vi "Add_Template.vi"(1 "X":dbl, 2 "Y":dbl) -> (0 "Output":dbl)   [LabVIEW 2013]
panel:
  # "Your code should take inputs X and Y and set output to the sum of X and Y"
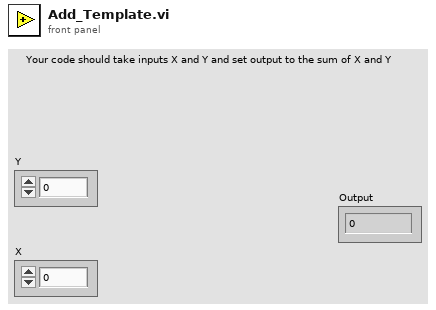
[diagram p1: front panel]
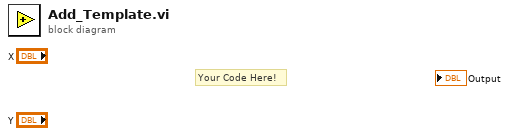
[diagram p0: block diagram]
diagram:
  # "Your Code Here!"
